vi "NI VeriStand - Get Channel Values by Block Data Reference.vi"(8 "error in (no error)":errorcluster, 10 "Values Array in":dbl[](array[numeric]), 11 "Block Data Ref":T1[](array[typedef]) {"Data Reference" format="%.0x"}) -> (0 "error out":errorcluster, 2 "Values Array out":dbl[](array[numeric]), 3 "Block Data Ref dup":T1[](array[typedef]) {"Data Reference" format="%.0x"})   [LabVIEW 2020, in "Custom Device API.lvlib"]
doc: "Returns the values of the inline custom device channels specified by <B>Block Data Ref</B>. You can use this VI to get multiple channel values at one time. Use the Get Channel Block Data References VI to get the channel data references for this VI.\n\nYou can use this VI in the Execute Model case of an Inline Model Interface custom device, or in the Read Data from HW or Write Data to HW cases of an Inline Hardware Interface custom device. Do not use this VI outside of an inline custom device."
uses:
  <vilib>/NI VeriStand/Custom Device API/Custom Device API.lvlib
  <vilib>/NI VeriStand/Custom Device API/Block Data Reference.ctl
  <vilib>/NI VeriStand/Custom Device API/Data Reference.ctl
  <vilib>/NI VeriStand/Custom Device API/Global Data Refs.vi
  <vilib>/NI VeriStand/Custom Device API/data/NIVeriStand_DataServices.dll
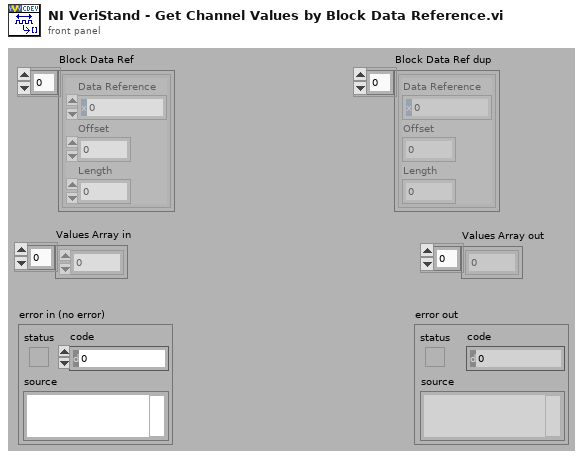
[diagram p1: front panel]
types:
  T1 = typedef "Custom Device API.lvlib/Block Data Reference.ctl" = cluster{"Data Reference":T2, "Offset":u64, "Length":u64}
  T2 = typedef "Custom Device API.lvlib/Data Reference.ctl" = i32
  T3 = typedef "Custom Device API.lvlib/Data Table Ref.ctl" = cluster{"Ptr.Beg":u64, "Ptr.End":u64}
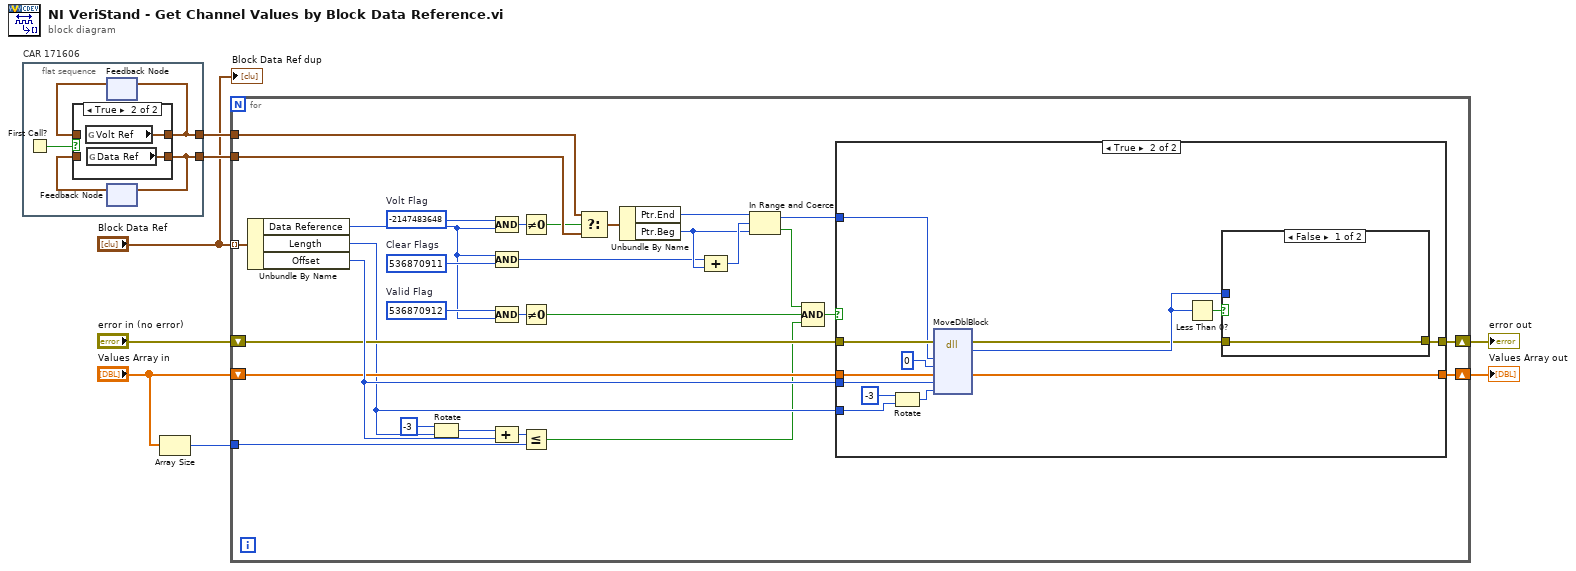
[diagram p0: block diagram]
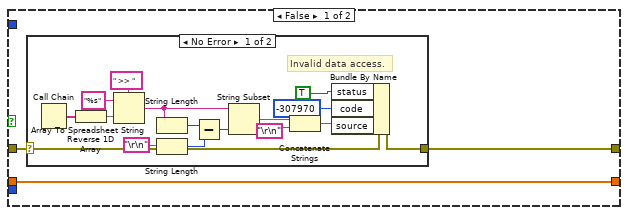
[diagram p3: hidden frame]
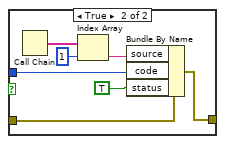
[diagram p5: hidden frame]
diagram:
  n1 = flat-sequence "CAR 171606" {
    tunnel: [w10] -> w3
    tunnel: [w9] -> w2
    frame #0 {
      n2 = First Call?() -> (First Call?: T/F=w13:bool)
      n3 = feedback #1() -> (w12:T3)  [unwired: 1 out]
      n4 = feedback #2() -> (w11:T3)  [unwired: 1 out]
      n5 = case shown="True" w13 {
        tunnel: [w15 w17] -> w10
        tunnel: w12 -> [w15 _]
        tunnel: [w14 w16] -> w9
        tunnel: w11 -> [w14 _]
        frame False {
        }
        frame True {
          n6 = global read "Global Data Refs.vi" "Volt Ref"() -> (w17:T3)
          n7 = global read "Global Data Refs.vi" "Data Ref"() -> (w16:T3)
        }
      }
      n8 = feedback-in #1(w10) -> ()
      n9 = feedback-in #2(w9) -> ()
    }
  }
  n10 = Array Size(array="Values Array in") -> (size(s)=w4:i32)
  n11 = for {
    tunnel: "Block Data Ref" -> [w30] mode=indexing
    shift-right: [w39] -> w8
    shift-left: "error in (no error)" -> [w40]
    tunnel: w3 -> [w26]
    tunnel: w2 -> [w46]
    shift-right: [w25] -> w6
    shift-left: "Values Array in" -> [w24]
    tunnel: w4 -> [w21]
    w32 = 536870912  # Valid Flag
    w34 = 536870911  # Clear Flags
    w37 = -2147483648  # Volt Flag
    n12 = Unbundle By Name(w30) -> ("Data Reference"=w27:T2, "Length"=w23:u64, "Offset"=w47:u64)
    n13 = Rotate(1:w23, 2:i8 -3 ("y")) -> (0:w19:u64)
    n14 = Compound Arithmetic op=AND(w37, w27) -> (w38:T2)
    n15 = Compound Arithmetic op=AND(w27, w34) -> (w28:T2)
    n16 = Compound Arithmetic op=AND(w32, w27) -> (w31:T2)
    n17 = Compound Arithmetic op=ADD(w19, w47) -> (w22:u64)
    n18 = Not Equal To 0?(x=w38) -> (x != 0?=w36:bool)
    n19 = Not Equal To 0?(x=w31) -> (x != 0?=w29:bool)
    n20 = Less Or Equal?(x=w22, y=w21) -> (x <= y?=w20:bool)
    n21 = Select(t=w26, s=w36, f=w46) -> (s? t:f=w35:T3)
    n22 = Unbundle By Name(w35) -> ("Ptr.End"=w42:u64, "Ptr.Beg"=w41:u64)
    n23 = Compound Arithmetic op=ADD(w28, w41) -> (w45:u64)
    n24 = In Range and Coerce(upper limit=w42, x=w45, lower limit=w41) -> (coerced(x)=w44:u64, In Range?=w43:bool)
    n25 = Compound Arithmetic op=AND(w43, w29, w20) -> (w33:bool)
    n26 = case shown="True" w33 {
      tunnel: w40 -> [w49 w80]
      tunnel: [w48 w68] -> w39
      tunnel: w44 -> [_ w76]
      tunnel: w23 -> [_ w72]
      tunnel: [w50 w78] -> w25
      tunnel: w24 -> [w50 w79]
      tunnel: w47 -> [_ w75]
      frame False {
        n27 = case shown="No Error" w49 {
          selector: w49 -> [w63 w67]
          tunnel: [w66 w67] -> w48
          frame No Error {
            # "Invalid data access."
            n28 = Call Chain() -> (call chain=w52:string[])
            n29 = Reverse 1D Array(array=w52) -> (reversed array=w59:string[])
            n30 = Array To Spreadsheet String(delimiter (Tab)=" >> ", array=w59, 3:"%s" ("format string")) -> (spreadsheet string=w60:string)
            n31 = String Length(string=w60) -> (length=w58:i32)
            n32 = String Length(string="\r\n") -> (length=w62:i32)
            n33 = Subtract(x=w58, y=w62) -> (x-y=w57:i32)
            n34 = String Subset(string=w60, length (rest)=w57) -> (substring=w53:string)  [unwired: 1 out]
            n35 = Concatenate Strings(w53, "\r\n") -> (w51:string)
            n36 = Bundle By Name(cluster=w63, "status"=TRUE, "code"=-307970, "source"=w51) -> (w66:errorcluster)
          }
          frame Error {
            # "Leave existing error."
          }
        }
      }
      frame True {
        n37 = Rotate(1:w72, 2:i8 -3 ("y")) -> (0:w73:u64)
        n38 = dll-call lib="e:/penguin/lvtoolchain/2020/eng32/export/20.0/20.0.0f11/win/vi.lib/NI VeriStand/Custom Device API/data/NIVeriStand_DataServices.*" fn="MoveDblBlock"(error in=w80, "srcPtr"=w76, "srcOffset"=u64 0, "dstPtr"=w79, "dstOffset"=w75, "count"=w73) -> (error out=w69:errorcluster, "return type"=w70:i32, "dstPtr"=w78:dbl[])  [unwired: 6 in, 1 out]
        n39 = Less Than 0?(x=w70) -> (x < 0?=w71:bool)
        n40 = case shown="False" w71 {
          tunnel: w70 -> [_ w84]
          tunnel: [w81 w86] -> w68
          tunnel: w69 -> [w81 w82]
          frame False {
          }
          frame True {
            n41 = Call Chain() -> (call chain=w87:string[])
            n42 = Index Array(array=w87, index=1) -> (element=w83:string)
            n43 = Bundle By Name(cluster=w82, "source"=w83, "code"=w84, "status"=TRUE) -> (w86:errorcluster)
          }
        }
      }
    }
  }
  "Values Array out" <- w6
  "error out" <- w8
  "Block Data Ref dup" <- "Block Data Ref"
